vi "fgv_DL950_buffer.vi"(7 "cmd":T2, 8 "error in":errorcluster, 11 "DL950 wfm 2":T1={"wfms"=[], "Waveform_2"={"t0"=0.0, "dt"=0.0, "Y"=[]}, "items"=[], "da950_array"=[10.0, 0.02, 0.074492, 0.033331, 0.018948904, 3.5928321, 0.0, 0.0, 400.375, 399.625, 3.5928321, 0.0, 0.0, 0.074492, 0.0, 0.0]}) -> (0 "error out":errorcluster, 3 "queue out":refnum<queue>)   [LabVIEW 2019]
uses:
  _ctrl/create-rw-close.ctl
  Durability/DL950_wfms.ctl
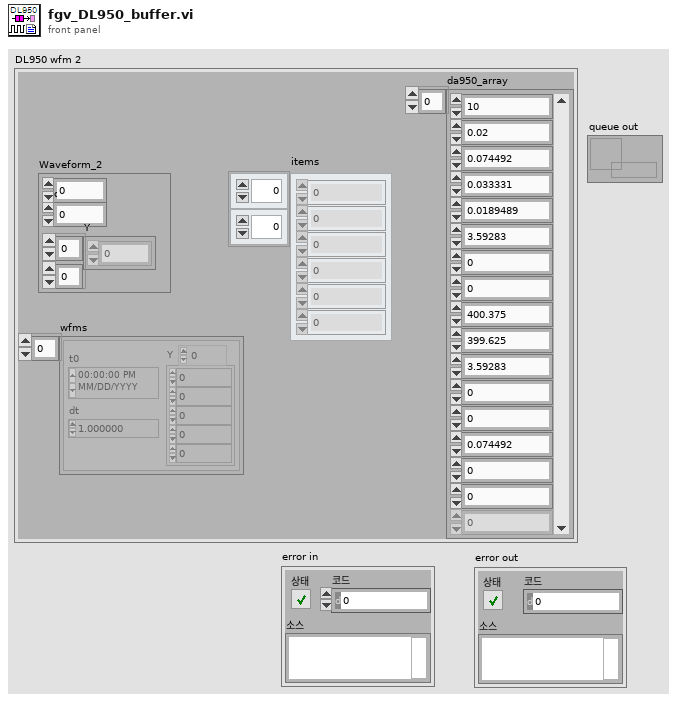
[diagram p1: front panel]
types:
  T1 = typedef "DL950_wfms.ctl" = cluster{"wfms":waveform(dbl)[], "Waveform_2":cluster{"t0":dbl, "dt":dbl, "Y":dbl[][]}, "items":dbl[][], "da950_array":dbl[]}
  T2 = typedef "create-rw-close.ctl" = enum16{"create", "write", "read", "delete", "close"}
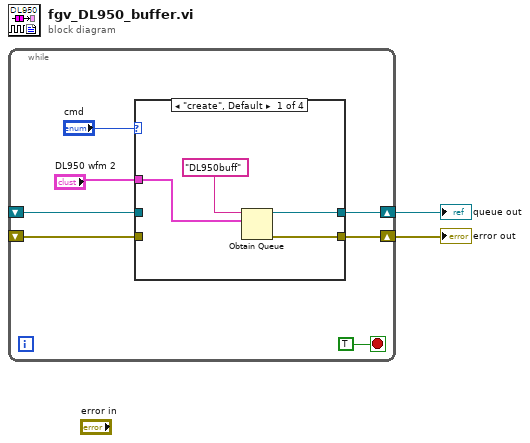
[diagram p0: block diagram]
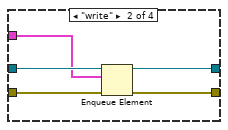
[diagram p2: hidden frame]
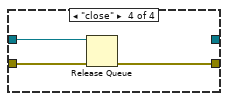
[diagram p4: hidden frame]
diagram:
  n1 = while {
    shift-right: [w7] -> w1
    shift-left: _ -> [w4]
    shift-right: [w6] -> w2
    shift-left: _ -> [w5]
    stop <- TRUE stop-if-true
    n2 = case shown="\"create\", Default" "cmd" {
      tunnel: [w13 w16 w20 _] -> w7
      tunnel: [w12 w17 w19 w22] -> w6
      tunnel: w5 -> [_ w18 w19 w23]
      tunnel: w4 -> [_ w15 w20 w21]
      tunnel: "DL950 wfm 2" -> [w10 w14 _ _]
      frame "create", Default {
        n3 = Obtain Queue(name (unnamed)="DL950buff" ("이름(이름없음)"), element data type=w10) -> (queue out=w13:refnum<queue>, error out=w12:errorcluster)  [unwired: 3 in, 1 out]
      }
      frame "write" {
        n4 = Enqueue Element(queue=w15, element=w14, error in (no error)=w18) -> (queue out=w16:refnum<queue>, error out=w17:errorcluster)  [unwired: 1 in, 1 out]
      }
      frame "read" {
      }
      frame "close" {
        n5 = Release Queue(queue=w21, error in (no error)=w23) -> (error out=w22:errorcluster)  [unwired: 1 in, 2 out]
      }
    }
  }
  "error out" <- w2
  "queue out" <- w1
